vi "Write CellBGKColorAlternate.vi"(8 "error in (no error)":errorcluster, 10 "CellBGKColorAlternate":u32(colorbox)=15790320, 11 "DataGridView in":refnum<class "DataGridView.lvclass">) -> (0 "error out":errorcluster, 3 "DataGridView out":refnum<class "DataGridView.lvclass">)   [LabVIEW 2014, in "DataGridView.lvclass"]
uses:
  DataGridView.lvclass
  System.Windows.Forms
  System.Drawing
  DataGridView.lvclass/DataGridView.ctl
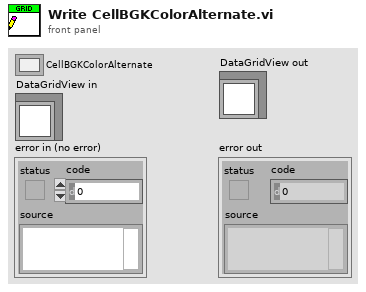
[diagram p1: front panel]
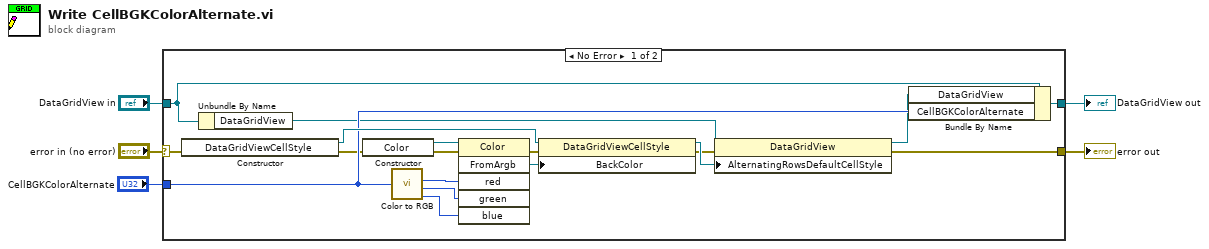
[diagram p0: block diagram]
diagram:
  n1 = case shown="No Error" "error in (no error)" {
    selector: "error in (no error)" -> [w9 w24]
    tunnel: [w7 w24] -> w4
    tunnel: [w23 w25] -> w2
    tunnel: "DataGridView in" -> [w12 w25]
    tunnel: "CellBGKColorAlternate" -> [w13 _]
    frame No Error {
      n2 = constructor class="DataGridViewCellStyle"(error in=w9) -> (reference out=w14:refnum<k24>, error out=w8:errorcluster)  [unwired: 2 in, 1 out]
      n3 = Unbundle By Name(w12) -> ("DataGridView"=w11:refnum<k24>)
      n4 = constructor class="Color"(error in=w8) -> (reference out=w16:refnum<k24>, error out=w17:errorcluster)  [unwired: 2 in, 1 out]
      n5 = call <vilib>:"Color to RGB.vi"("Color"=w13) -> ("R"=w20:u8, "G"=w21:u8, "B"=w22:u8)  [unwired: 1 out]
      n6 = invoke class="Color" method="FromArgb"(reference=w16, error in=w17, "red"=w20, "green"=w21, "blue"=w22) -> (error out=w18:errorcluster, "FromArgb"=w19:refnum<k24>)  [unwired: 1 in, 4 out]
      n7 = property class="DataGridViewCellStyle"(reference=w14, error in=w18, "BackColor"=w19) -> (reference out=w15:refnum<k24>, error out=w10:errorcluster)
      n8 = property class="DataGridView"(reference=w11, error in=w10, "AlternatingRowsDefaultCellStyle"=w15) -> (reference out=w6:refnum<k24>, error out=w7:errorcluster)
      n9 = Bundle By Name(cluster=w12, "DataGridView"=w6, "CellBGKColorAlternate"=w13) -> (w23:refnum<class "DataGridView.lvclass">)
    }
    frame Error {
    }
  }
  "error out" <- w4
  "DataGridView out" <- w2
